vi "Apply Motor Config Obj by Label.vi"(8 "error in (no error)":errorcluster, 10 "Motor Configuration Obj":refnum<class "Motor Configuration.lvclass">, 11 "Motions Configuration in":refnum<class "Motions Configuration.lvclass">) -> (0 "error out":errorcluster, 3 "Motions Configuration out":refnum<class "Motions Configuration.lvclass">)   [LabVIEW 2016, in "Hardware.lvlib" / "Motions.lvlib" / "Motions Configuration.lvclass"]
uses:
  <userlib>/Common Components/Hardware/Abstract System/Motions/Motions Config/Motions Configuration.lvclass
  <userlib>/Common Components/Hardware/Motor/Motor Config/Motor Configuration.lvclass
  <userlib>/Common Components/Hardware/Abstract System/Motions/Motions Config/Motions Configuration.lvclass/Motions Configuration.ctl
  <userlib>/Common Components/Hardware/Abstract System/Motions/Motions/Motions.lvclass/Motions.ctl
  <userlib>/Common Components/Hardware/Abstract Hardware/Hardware.lvclass/Hardware.ctl
  <userlib>/Common Components/Hardware/Abstract Hardware/Read Label.vi
  <userlib>/Common Components/Hardware/Motor/Motor/Motor.lvclass
  C:/Program Files (x86)/National Instruments/LabVIEW 2016/user.lib/Common Components/Hardware/Abstract Hardware/Hardware.lvclass
  <userlib>/Common Components/Hardware/Abstract System/Motions/Motions/Motions.lvclass
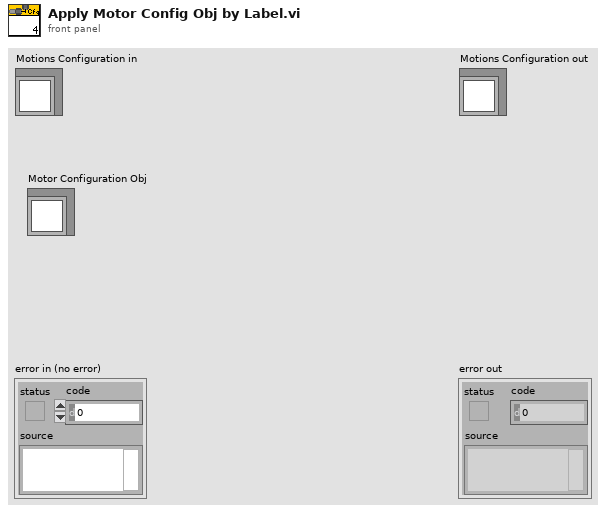
[diagram p1: front panel]
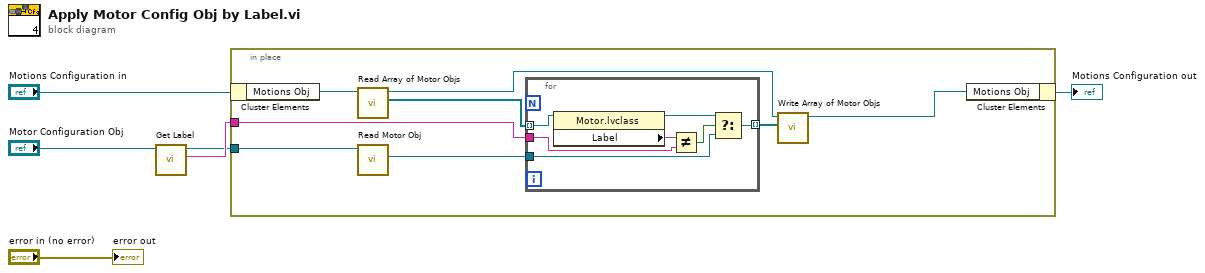
[diagram p0: block diagram]
diagram:
  n1 = call <userlib>:"Get Label.vi"("Motor Configuration in"="Motor Configuration Obj") -> ("Label"=w2:string, "Motor Configuration out"=w1:refnum<class "Motor Configuration.lvclass">)  [unwired: 8 in, 1 out]
  n2 = in-place {
    in-place-border: w2 -> [w14]
    in-place-border: w1 -> [w13]
    n3 = in-place-cluster #1("Motions Configuration in") -> ("Motions Obj"=w12:refnum<class "Motions.lvclass">)
    n4 = call <userlib>:"Read Array of Motor Objs.vi"("Motions in"=w12) -> ("Array of Motor Objs"=w10:refnum<class "Motor.lvclass">[], "Motions out"=w7:refnum<class "Motions.lvclass">)  [unwired: 9 in]
    n5 = call <userlib>:"Read Motor Obj.vi"("Motor Configuration in"=w13) -> ("Hardware.lvlib:Motor.lvlib:Motor.lvclass"=w9:refnum<class "Motor.lvclass">)  [unwired: 8 in, 2 out]
    n6 = for {
      tunnel: w10 -> [w21] mode=indexing
      tunnel: w14 -> [w20]
      tunnel: w9 -> [w17]
      tunnel: [w16] -> w11 mode=indexing
      n7 = property class="Motor.lvclass"(reference=w21) -> (reference out=w18:refnum<class "Motor.lvclass">, "Label"=w15:string)  [unwired: 1 in, 1 out]
      n8 = Not Equal?(x=w15, y=w20) -> (x != y?=w19:bool)
      n9 = Select(t=w18, s=w19, f=w17) -> (s? t:f=w16:refnum<class "Motor.lvclass">)
    }
    n10 = call <userlib>:"Write Array of Motor Objs.vi"("Array of Motor Objs"=w11, "Motions in"=w7) -> ("Motions out"=w8:refnum<class "Motions.lvclass">)  [unwired: 9 in]
    n11 = in-place-cluster #1("Motions Obj"=w8) -> (→"Motions Configuration out":refnum<class "Motions Configuration.lvclass">)
  }
  "error out" <- "error in (no error)"
